vi "Unflatten U64.vi"(3 "Flat Data":u8[](array[numeric]) format="%.0x", 4 "Endian":T1) -> (5 "U64":u64)   [LabVIEW 2021, in "DataTypes_CIF_U.lvlib"]
uses:
  DataTypes_CIF_U.lvlib
  Endian.ctl
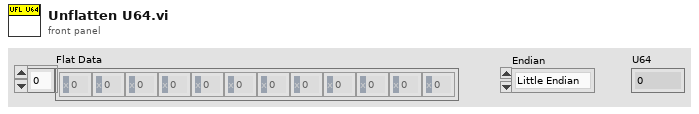
[diagram p1: front panel]
types:
  T1 = typedef "DataTypes_CIF_U.lvlib/Endian.ctl" = enum16{"Little Endian", "Big Endian"}
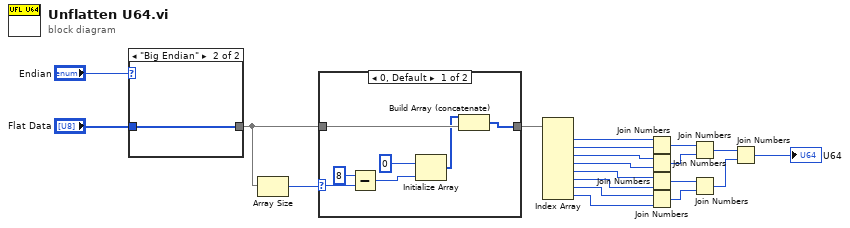
[diagram p0: block diagram]
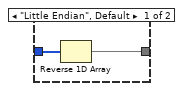
[diagram p3: hidden frame]
diagram:
  n1 = case shown="\"Big Endian\"" "Endian" {
    tunnel: "Flat Data" -> [w22 w23]
    tunnel: [w21 w23] -> w4
    frame "Little Endian", Default {
      n2 = Reverse 1D Array(array=w22) -> (reversed array=w21:u8[])
    }
    frame "Big Endian" {
    }
  }
  n3 = Array Size(array=w4) -> (size(s)=w6:i32)
  n4 = case shown="0, Default" w6 {
    selector: w6 -> [w30 _]
    tunnel: w4 -> [w26 w31]
    tunnel: [w24 w31] -> w5
    frame 0, Default {
      n5 = Subtract(x=8, y=w30) -> (x-y=w27:i32)
      n6 = Initialize Array(u8 0 ("element"), w27) -> (w25:u8[])
      n7 = Build Array (concatenate)(w25, w26) -> (w24:u8[])
    }
    frame 8.. {
    }
  }
  n8 = Index Array(array=w5) -> (element #1=w20:u8, element #2=w13:u8, element #3=w12:u8, element #4=w11:u8, element #5=w10:u8, element #6=w9:u8, element #7=w8:u8, element #8=w7:u8)  [unwired: 8 in]
  n9 = Join Numbers(hi=w20, lo=w13) -> ((hi.lo)=w19:u16)
  n10 = Join Numbers(hi=w12, lo=w11) -> ((hi.lo)=w15:u16)
  n11 = Join Numbers(hi=w10, lo=w9) -> ((hi.lo)=w17:u16)
  n12 = Join Numbers(hi=w8, lo=w7) -> ((hi.lo)=w14:u16)
  n13 = Join Numbers(hi=w19, lo=w15) -> ((hi.lo)=w18:u32)
  n14 = Join Numbers(hi=w17, lo=w14) -> ((hi.lo)=w16:u32)
  n15 = Join Numbers(hi=w18, lo=w16) -> ((hi.lo)=→"U64":u64)
